vi "Configure HSDIO_SuBUS.vi"(8 "error in (no error)":errorcluster, 11 "HDSIO_Settings":T2={"HSDIO VISA"="6556_0", "logic family "=8, "Clock Rate"=20000000.0, "channel list (Clock,Data)"="0"} {"Clock Rate" format="%.2p"; "logic family" items=["5.0V Logic"=5, "3.3V Logic"=6, "2.5V Logic"=7, "1.8V Logic"=8, "1.5V Logic"=80, "1.2V Logic"=81]}) -> (0 "error out":errorcluster, 2 "HDSIO_Settings 2":T2={"HSDIO VISA"="6556_0", "logic family "=8, "Clock Rate"=20000000.0, "channel list (Clock,Data)"="0"} {"Clock Rate" format="%.2p"; "logic family" items=["5.0V Logic"=5, "3.3V Logic"=6, "2.5V Logic"=7, "1.8V Logic"=8, "1.5V Logic"=80, "1.2V Logic"=81]}, 3 "HSDIO Sessions":T3)   [LabVIEW 2013]
uses:
  <instrlib>/niHSDIO/niHSDIO.llb/niHSDIO_ctl Voltage Logic Family Values (Ring).ctl
  <instrlib>/niHSDIO/niHSDIO.llb/niHSDIO_ctl Generation Mode Values (Ring).ctl
  <instrlib>/niHSDIO/niHSDIO.llb/niHSDIO_ctl Data Position Values (Ring).ctl
  <instrlib>/niHSDIO/niHSDIO.llb/niHSDIO_ctl Trigger Source Values (Ring).ctl
  <instrlib>/niHSDIO/niHSDIO.llb/niHSDIO_ctl Exported Signal Name Values (Ring).ctl
  <instrlib>/niHSDIO/niHSDIO.llb/niHSDIO Configure Data Voltage Logic Family.vi
  <instrlib>/niHSDIO/niHSDIO.llb/niHSDIO Configure Initial State (String).vi
  <instrlib>/niHSDIO/niHSDIO.llb/niHSDIO Configure Idle State (String).vi
  <instrlib>/niHSDIO/niHSDIO.llb/niHSDIO Configure Digital Edge Start Trigger.vi
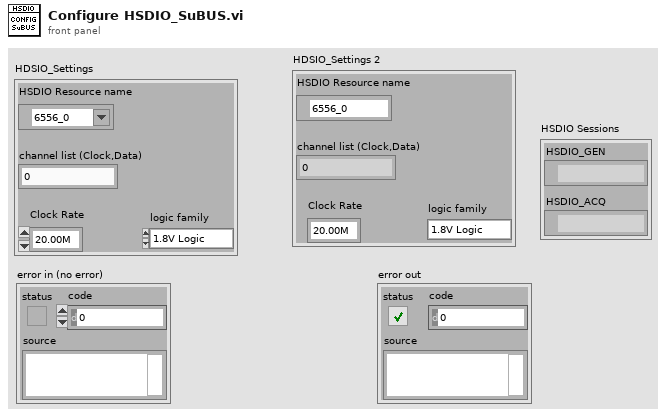
[diagram p1: front panel]
types:
  T1 = typedef "niHSDIO_ctl Voltage Logic Family Values (Ring).ctl" = i32
  T2 = cluster{"HSDIO VISA":refnum<k15>, "logic family ":T1, "Clock Rate":dbl, "channel list (Clock,Data)":string}
  T3 = cluster{"HSDIO_ACQ":refnum<k15>, "HSDIO_GEN":refnum<k15>}
  T4 = typedef "niHSDIO_ctl Exported Signal Name Values (Ring).ctl" = u16
  T5 = typedef "niHSDIO_ctl Trigger Source Values (Ring).ctl" = string
  T6 = typedef "niHSDIO_ctl Data Position Values (Ring).ctl" = i32
  T7 = typedef "niHSDIO_ctl Generation Mode Values (Ring).ctl" = i32
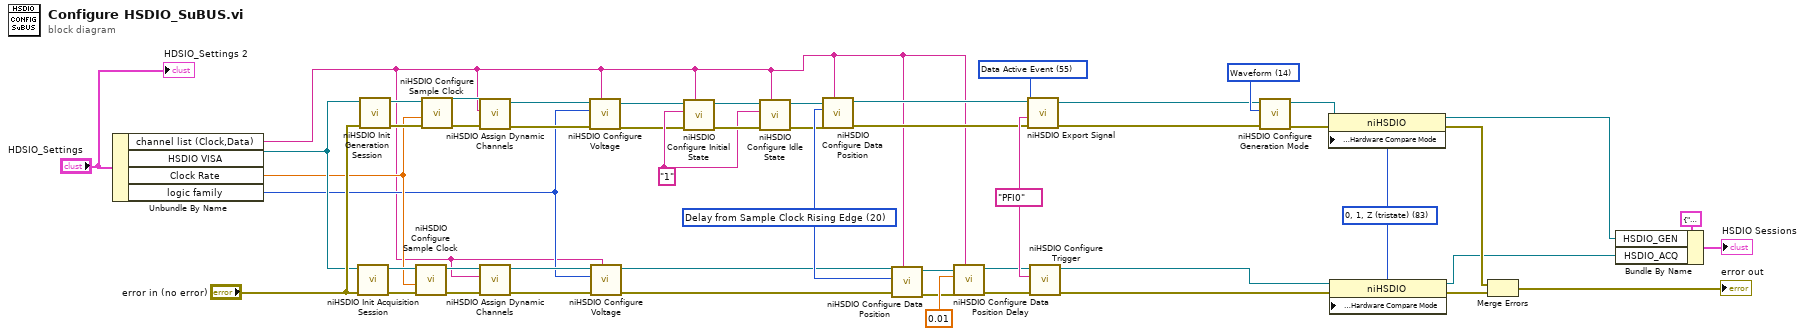
[diagram p0: block diagram]
diagram:
  w34 = "1" ("initial state")
  w42 = T4 55 items=["Sample Clock"=51, "Reference Clock"=52, "Start Trigger"=53, "Reference Trigger"=54, "Advance Trigger"=61, "Pause Trigger"=57, "Script Trigger"=58, "Stop Trigger"=82, "Data Active Event"=55, "Marker Event"=59, "Ready For Start Event"=56, "Ready For Advance Event"=66, "End Of Record Event"=68, "Onboard Ref Clock"=60] ("signal (sample clock)")
  w41 = T5 "PFI0" ("source (PFI 0)")
  w47 = 83 items=["0, 1 (binary)"=77, "0, 1, Z (tristate)"=83, "0, 1, Z, L, H, X (stim/resp)"=78, "L, H, X (resp only)"=79] ("Advanced:Supported Data States")
  w46 = T6 20 items=["Sample Clock Rising Edge"=18, "Sample Clock Falling Edge"=19, "Delay from Sample Clock Rising Edge"=20] ("position (rising edge)")
  w50 = T7 14 items=["Waveform"=14, "Scripted"=15] ("generation mode (waveform)")
  n1 = Unbundle By Name("HDSIO_Settings") -> ("channel list (Clock,Data)"=w6:string, "HSDIO VISA"=w12:refnum<k15>, "Clock Rate"=w11:dbl, "logic family"=w10:T1)
  n2 = call <instrlib>:"niHSDIO Init Acquisition Session.vi"("error in (no error)"="error in (no error)", "resource name"=w12) -> ("error out"=w33:errorcluster, "instrument handle out"=w37:refnum<k15>)  [unwired: 8 in]
  n3 = call <instrlib>:"niHSDIO Init Generation Session.vi"("error in (no error)"="error in (no error)", "resource name"=w12) -> ("error out"=w36:errorcluster, "instrument handle out"=w38:refnum<k15>)  [unwired: 8 in]
  n4 = call <instrlib>:"niHSDIO Configure Sample Clock.vi"("error in (no error)"=w33, "clock rate (50MHz)"=w11, "instrument handle"=w37) -> ("error out"=w49:errorcluster, "instrument handle out"=w48:refnum<k15>)  [unwired: 7 in]
  n5 = call <instrlib>:"niHSDIO Configure Sample Clock.vi"("error in (no error)"=w36, "clock rate (50MHz)"=w11, "instrument handle"=w38) -> ("error out"=w52:errorcluster, "instrument handle out"=w51:refnum<k15>)  [unwired: 7 in]
  n6 = call <instrlib>:"niHSDIO Assign Dynamic Channels.vi"("error in (no error)"=w52, "channel list (all:\"\")"=w6, "instrument handle"=w51) -> ("error out"=w32:errorcluster, "instrument handle out"=w31:refnum<k15>)  [unwired: 7 in]
  n7 = call <instrlib>:"niHSDIO Assign Dynamic Channels.vi"("error in (no error)"=w49, "channel list (all:\"\")"=w6, "instrument handle"=w48) -> ("error out"=w30:errorcluster, "instrument handle out"=w29:refnum<k15>)  [unwired: 7 in]
  n8 = call-poly <instrlib>:"niHSDIO Configure Voltage.vi"("channel list (all:\"\")"=w6, "error in (no error)"=w32, "logic family (3.3V logic)"=w10, "instrument handle"=w31) -> ("error out"=w28:errorcluster, "instrument handle out"=w27:refnum<k15>)  [unwired: 6 in]
  n9 = call-poly <instrlib>:"niHSDIO Configure Voltage.vi"("channel list (all:\"\")"=w6, "error in (no error)"=w30, "logic family (3.3V logic)"=w10, "instrument handle"=w29) -> ("error out"=w24:errorcluster, "instrument handle out"=w23:refnum<k15>)  [unwired: 6 in]
  n10 = call-poly <instrlib>:"niHSDIO Configure Initial State.vi"("channel list"=w6, "error in (no error)"=w28, "initial state"=w34, "instrument handle"=w27) -> ("error out"=w40:errorcluster, "instrument handle out"=w39:refnum<k15>)  [unwired: 6 in]
  n11 = call-poly <instrlib>:"niHSDIO Configure Idle State.vi"("channel list"=w6, "error in (no error)"=w40, "idle state"=w34, "instrument handle"=w39) -> ("error out"=w26:errorcluster, "instrument handle out"=w25:refnum<k15>)  [unwired: 6 in]
  n12 = call <instrlib>:"niHSDIO Configure Data Position.vi"("channel list (all:\"\")"=w6, "error in (no error)"=w26, "position (rising edge)"=w46, "instrument handle"=w25) -> ("error out"=w22:errorcluster, "instrument handle out"=w21:refnum<k15>)  [unwired: 6 in]
  n13 = call <instrlib>:"niHSDIO Configure Data Position.vi"("channel list (all:\"\")"=w6, "error in (no error)"=w24, "position (rising edge)"=w46, "instrument handle"=w23) -> ("error out"=w43:errorcluster, "instrument handle out"=w44:refnum<k15>)  [unwired: 6 in]
  n14 = call <instrlib>:"niHSDIO Configure Data Position Delay.vi"("channel list (all:\"\")"=w6, "error in (no error)"=w43, "delay (0.000)"=0.01, "instrument handle"=w44) -> ("error out"=w20:errorcluster, "instrument handle out"=w19:refnum<k15>)  [unwired: 6 in]
  n15 = call <instrlib>:"niHSDIO Export Signal.vi"("error in (no error)"=w22, "output terminal (do not export)"=w41, "signal (sample clock)"=w42, "instrument handle"=w21) -> ("error out"=w2:errorcluster, "instrument handle out"=w1:refnum<k15>)  [unwired: 6 in]
  n16 = call-poly <instrlib>:"niHSDIO Configure Trigger.vi"("error in (no error)"=w20, "source (PFI 0)"=w41, "instrument handle"=w19) -> ("error out"=w18:errorcluster, "instrument handle out"=w17:refnum<k15>)  [unwired: 7 in]
  n17 = call <instrlib>:"niHSDIO Configure Generation Mode.vi"("error in (no error)"=w2, "generation mode (waveform)"=w50, "instrument handle"=w1) -> ("error out"=w16:errorcluster, "instrument handle out"=w15:refnum<k15>)  [unwired: 7 in]
  n18 = property on="Property Node" class="niHSDIO"(reference=w15, error in=w16, "Advanced:Hardware Compare:Hardware Compare Mode"=w47) -> (reference out=w3:refnum<k15>, error out=w13:errorcluster)
  n19 = property on="Property Node" class="niHSDIO"(reference=w17, error in=w18, "Advanced:Hardware Compare:Hardware Compare Mode"=w47) -> (reference out=w8:refnum<k15>, error out=w14:errorcluster)
  n20 = Merge Errors(w13, w14) -> (→"error out":errorcluster)
  n21 = Bundle By Name(cluster=T3 {"HSDIO_ACQ"="", "HSDIO_GEN"=""} ("HSDIO Sessions"), "HSDIO_GEN"=w3, "HSDIO_ACQ"=w8) -> (→"HSDIO Sessions":T3)
  "HDSIO_Settings 2" <- "HDSIO_Settings"
